vi "Read size.vi"(8 "error in (no error)":errorcluster, 11 "Wire in":refnum<class "Decoration.lvclass">) -> (0 "error out":errorcluster, 2 "size":T1, 3 "Wire out":refnum<class "Decoration.lvclass">)   [LabVIEW 2023, in "TLC_Scripto.lvlib" / "Decoration.lvclass"]
uses:
  Decoration.lvclass
  <vilib>/Utility/miscctls.llb/LVBoundsTypeDef.ctl
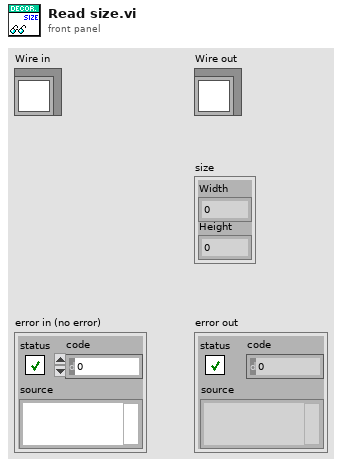
[diagram p1: front panel]
types:
  T1 = typedef "LVBoundsTypeDef.ctl" = cluster{"Width":u32, "Height":u32}
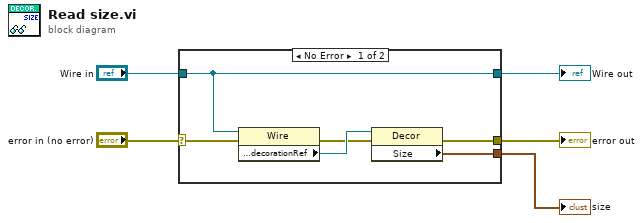
[diagram p0: block diagram]
diagram:
  n1 = case shown="No Error" "error in (no error)" {
    selector: "error in (no error)" -> [w8 w13]
    tunnel: [w7 w13] -> w4
    tunnel: [w11 w12] -> w2
    tunnel: "Wire in" -> [w11 w12]
    tunnel: [w6 _] -> w1
    frame No Error {
      n2 = property class="Wire"(reference=w11, error in=w8) -> (error out=w9:errorcluster, "Properties:decorationRef"=w10:refnum<vi>)  [unwired: 1 out]
      n3 = property class="Decor"(reference=w10, error in=w9) -> (error out=w7:errorcluster, "Size"=w6:T1)  [unwired: 1 out]
    }
    frame Error {
    }
  }
  "error out" <- w4
  "Wire out" <- w2
  "size" <- w1
